vi "q_update.vi"(0 "output valid 42":bool, 1 "K22":fxp<+,32,16>, 2 "K11":fxp<+,32,16>, 3 "output valid 22":bool, 4 "output valid 11":bool, 6 "K42":fxp<+,32,16>, 7 "Q1_temp off":fxp<+/-,32,16>, 8 "output valid 31":bool, 9 "Q2_temp off":fxp<+/-,32,16>, 10 "K31":fxp<+,32,16>) -> (12 "Q1_temp":fxp<+/-,32,16>, 13 "q4_ready":bool, 14 "q1_ready":bool, 15 "Q2_temp":fxp<+/-,32,16>, 16 "q2_ready":bool, 17 "Q3_temp":fxp<+/-,32,16>, 18 "q3_ready":bool, 19 "Q4_update":fxp<+/-,32,16>)   [LabVIEW 2020]
uses:
  <vilib>/rvi/FXPMathLib/FxpMul/XNode/nifxpmath_Multiplier.xnode
  <vilib>/rvi/FXPMathLib/sim/FxpSim.dll
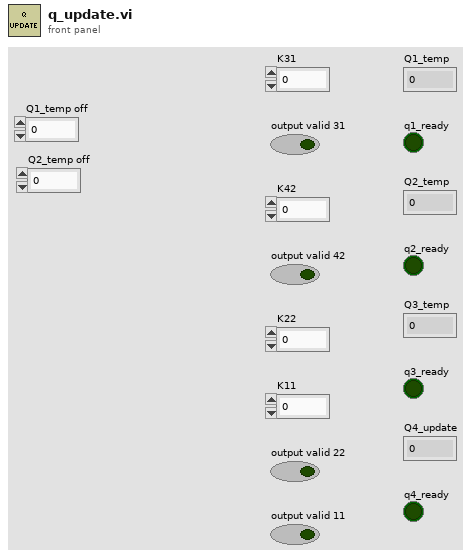
[diagram p1: front panel]
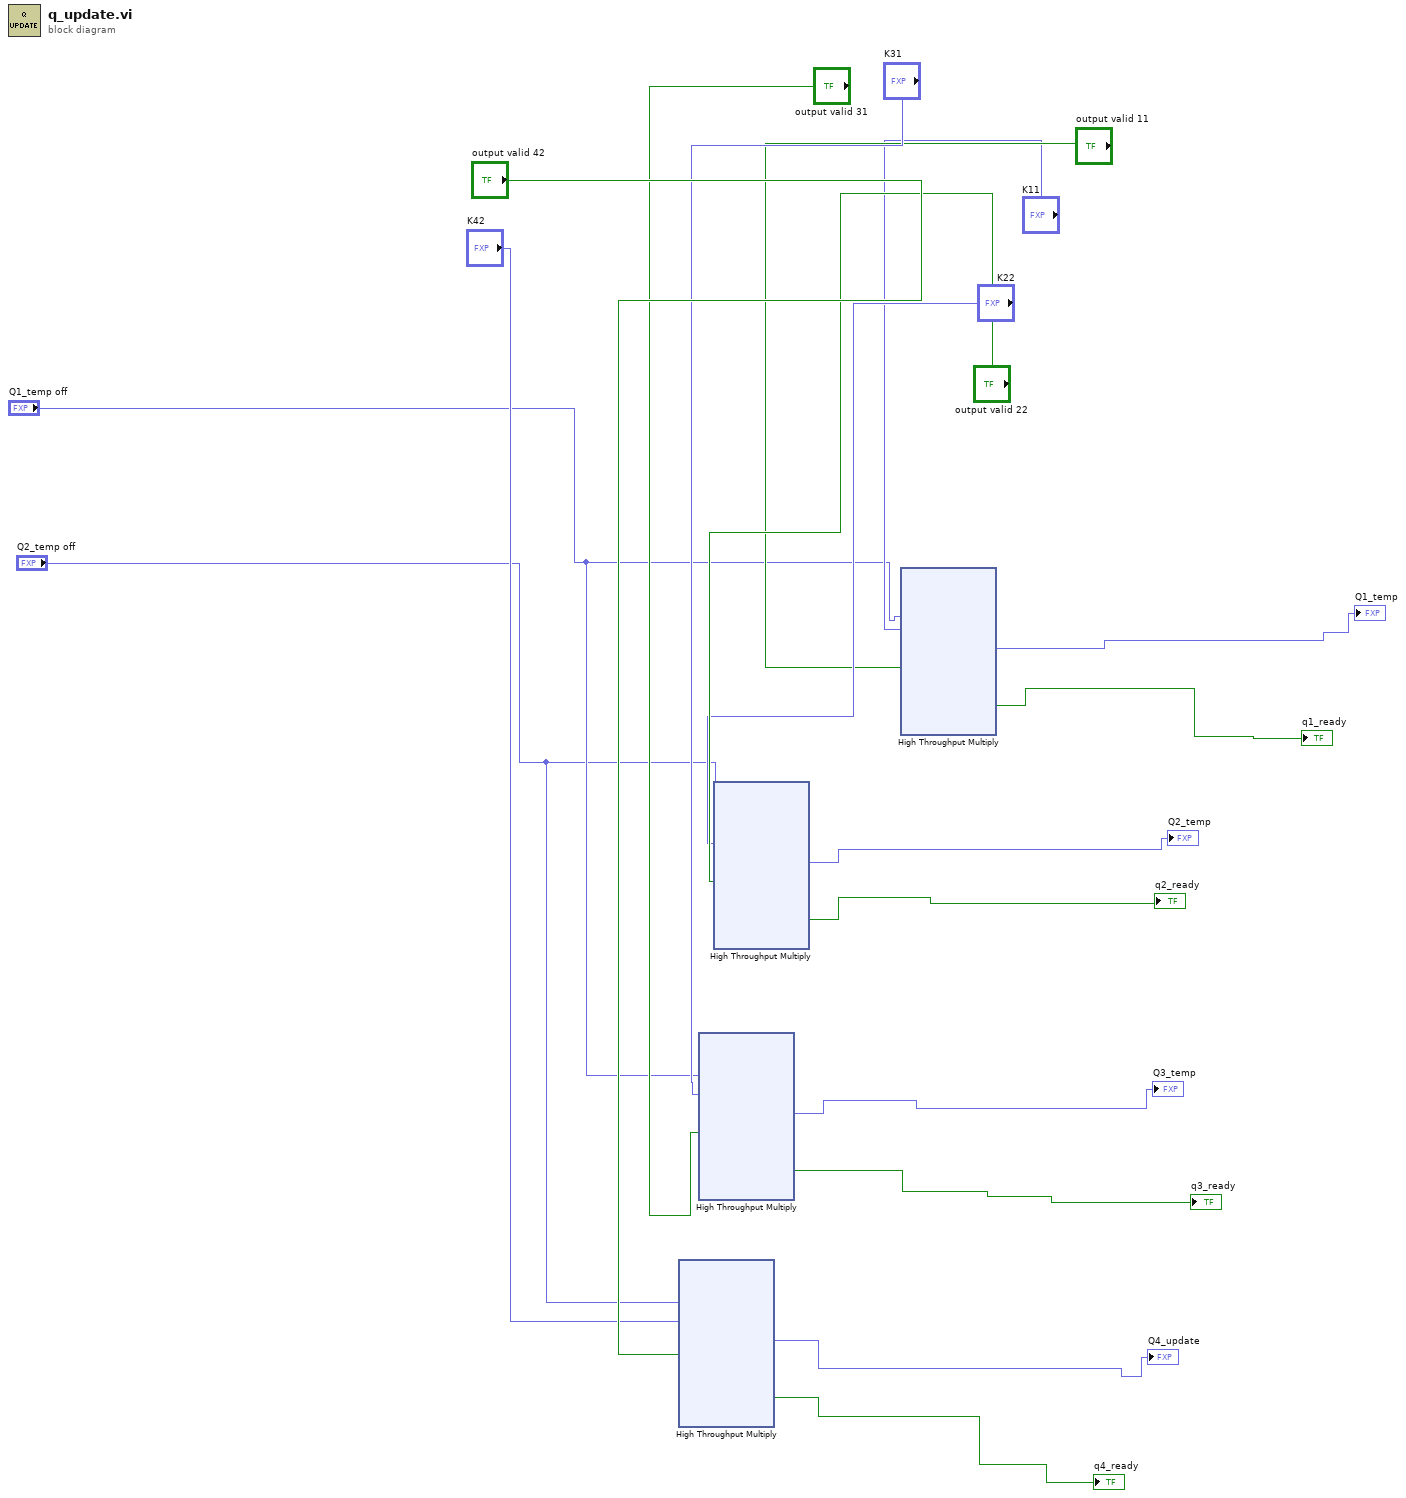
[diagram p0: block diagram]
diagram:
  n1 = xnode "High Throughput Multiply"("x"="Q2_temp off", "y"="K42", "input valid"="output valid 42") -> ("x*y"=→"Q4_update":fxp<+/-,32,16>, "output valid"=→"q4_ready":bool)  [unwired: 1 in, 1 out]
  n2 = xnode "High Throughput Multiply"("x"="Q1_temp off", "y"="K31", "input valid"="output valid 31") -> ("x*y"=→"Q3_temp":fxp<+/-,32,16>, "output valid"=→"q3_ready":bool)  [unwired: 1 in, 1 out]
  n3 = xnode "High Throughput Multiply"("x"="Q2_temp off", "y"="K22", "input valid"="output valid 22") -> ("x*y"=→"Q2_temp":fxp<+/-,32,16>, "output valid"=→"q2_ready":bool)  [unwired: 1 in, 1 out]
  n4 = xnode "High Throughput Multiply"("x"="Q1_temp off", "y"="K11", "input valid"="output valid 11") -> ("x*y"=→"Q1_temp":fxp<+/-,32,16>, "output valid"=→"q1_ready":bool)  [unwired: 1 in, 1 out]
